vi "Write Master.vi"(8 "error in":errorcluster, 11 "TeleOp Data in":T1) -> (0 "error out":errorcluster, 3 "TeleOp Data out":T1)   [LabVIEW 2018]
uses:
  TypeDefs/Teleop Data Cluster.ctl
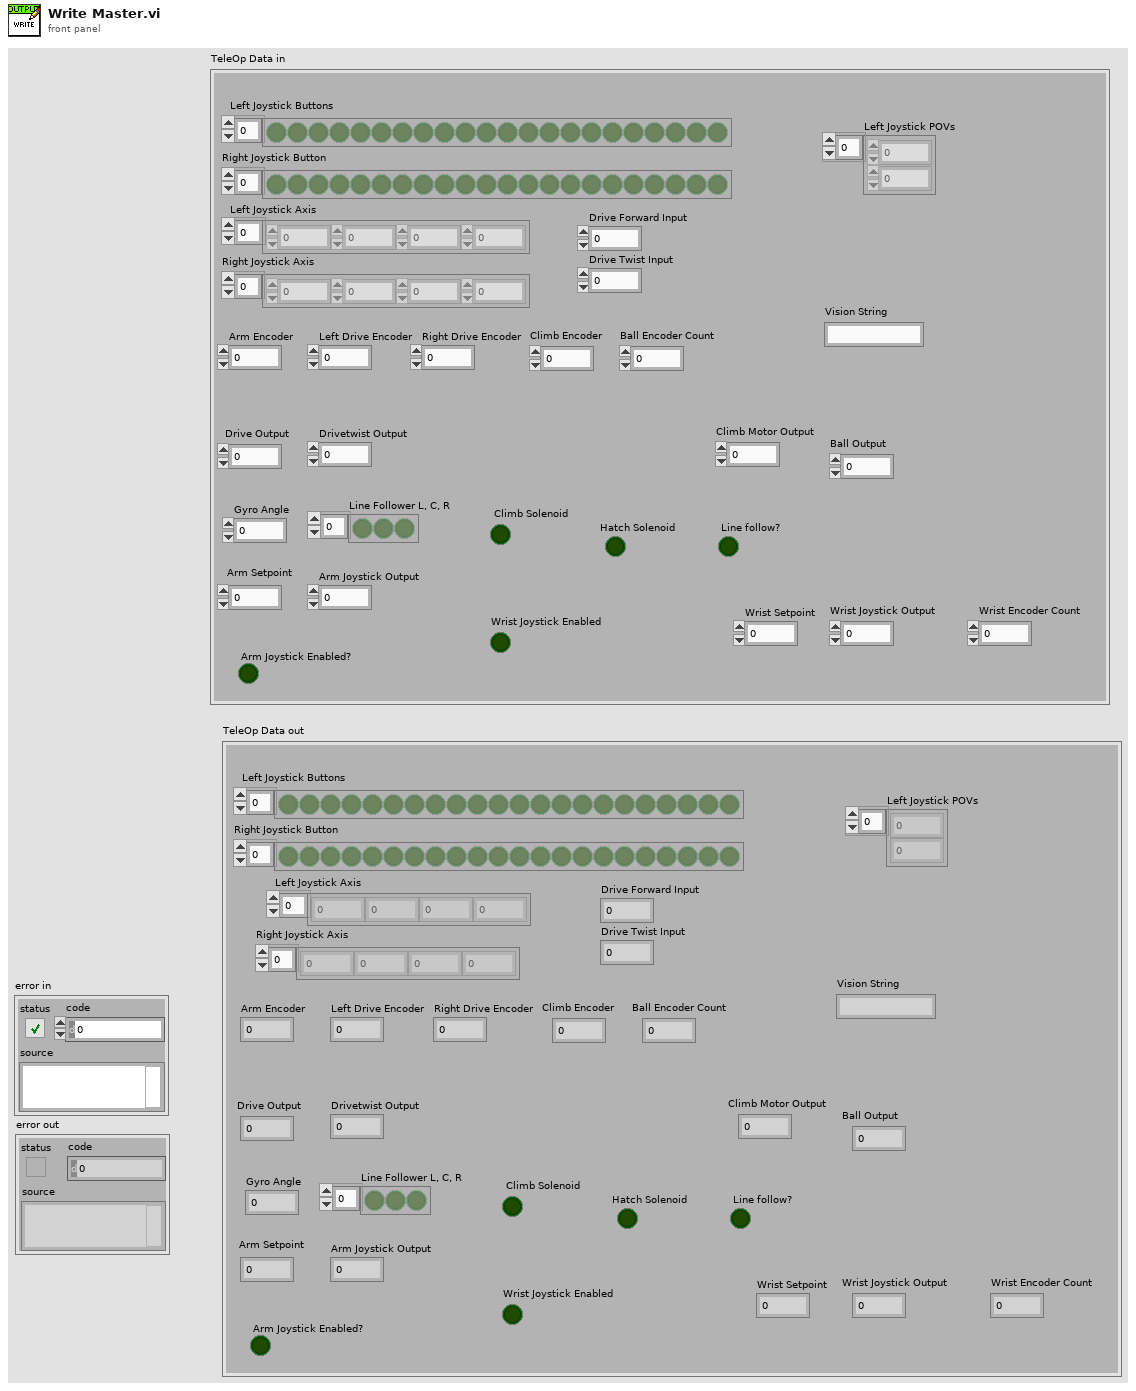
[diagram p1: front panel]
types:
  T1 = typedef "Teleop Data Cluster.ctl" = cluster{"Drive Forward Input ":dbl, "Drive Twist Input":dbl, "Drive Output":dbl, "Drivetwist Output":dbl, "Left Joystick Buttons":bool[], "Left Joystick Axis":dbl[], "Right Joystick Axis":dbl[], "Right Joystick Button":bool[], "Arm Encoder":dbl, "Left Drive Encoder":dbl, "Right Drive Encoder":dbl, "Gyro Angle ":dbl, "Arm Joystick Output  ":dbl, "Line Follower L, C, R ":bool[], "Line follow?":bool, " Climb Solenoid":bool, "Wrist Encoder Count":dbl, "Wrist Joystick Output":dbl, "Ball Encoder Count":dbl, "Ball Output":dbl, "Climb Encoder":dbl, "Climb Motor Output":dbl, " Hatch Solenoid":bool, "Arm Setpoint ":dbl, "Wrist Setpoint ":dbl, "Arm Joystick Enabled?":bool, "Wrist Joystick Enabled":bool, "Vision String":string, "Left Joystick POVs":i16[]}
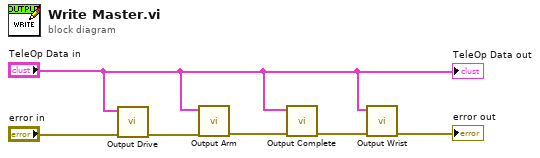
[diagram p0: block diagram]
diagram:
  n1 = call "Output Drive.vi"("error in (no error)"="error in", "TeleOp Data Cluster"="TeleOp Data in") -> ("error out"=w2:errorcluster)  [unwired: 9 in]
  n2 = call "Output Arm.vi"("error in (no error)"=w2, "TeleOp Data Cluster"="TeleOp Data in") -> ("error out"=w1:errorcluster)  [unwired: 9 in]
  n3 = call "Output Complete.vi"("error in  2"=w1, "TeleOp Data Cluster 2"="TeleOp Data in") -> ("error out  2"=→"error out":errorcluster)  [unwired: 9 in]
  n4 = call "Output Wrist.vi"("TeleOp Data Cluster"="TeleOp Data in") -> ()  [unwired: 11 in]
  "TeleOp Data out" <- "TeleOp Data in"
